vi "Emballage_BDD_CreationRapportParCarton_Modele.vi"(8 "error in (no error)":errorcluster caption="entrée d'erreur (pas d'erreur)", 11 "N° Cmd":string) -> (0 "error out":errorcluster caption="sortie d'erreur", 2 "chemin complet":path)   [LabVIEW 2020]
doc: "Envoi un mail avec la liste des valves emballées en pièce jointe si spécifié dans le fichier XML PP de la valve (FlatProp) ou correspondance produit code barre.txt (autres valves)"
uses:
  Modules/FS/60_FS_Controles/60_FS_SetGet.ctl
panel:
  out "temps Exe [s] 1":dbl
  out "temps Exe [s]":dbl
  out "Liste n° pièces de la cmde":string[](array[string])
  out "Carton":string[](array[string])
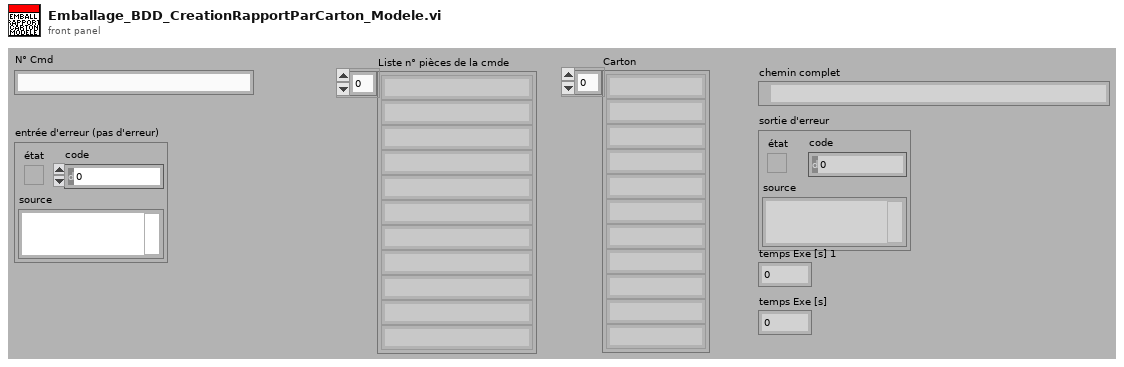
[diagram p1: front panel]
types:
  T1 = typedef "60_FS_SetGet.ctl" = enum16{"set", "get"}
  T2 = typedef "DATA commande.ctl" = cluster{"n°article FAS":string, "n° cmde FAS":string, "quantité cmde":string, "ID LIG cmde":string, "n° cmde client":string, "nom client":string, "n° article client":string, "indice revision client":string, "société de facturation":string, "langue a utiliser":string}
  T3 = cluster{"Admin-réseau":path, "XML-Réseau":path, " Résultat tests-Réseau":path, " Archive prôbleme-Réseau":path, " Archive Test  Local":path}
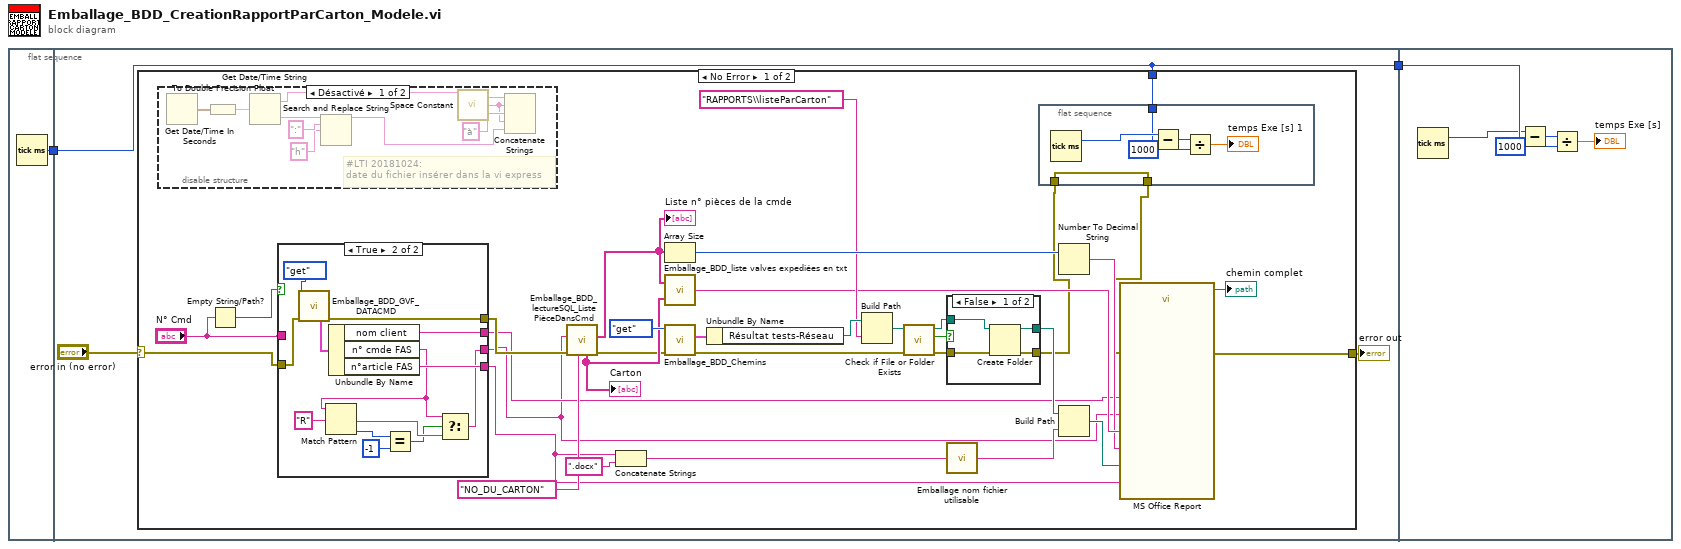
[diagram p0: block diagram]
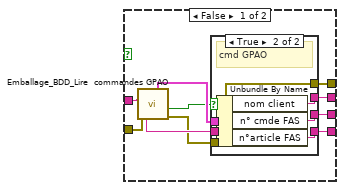
[diagram p2: hidden frame]
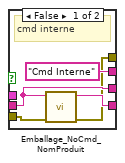
[diagram p3: hidden frame]
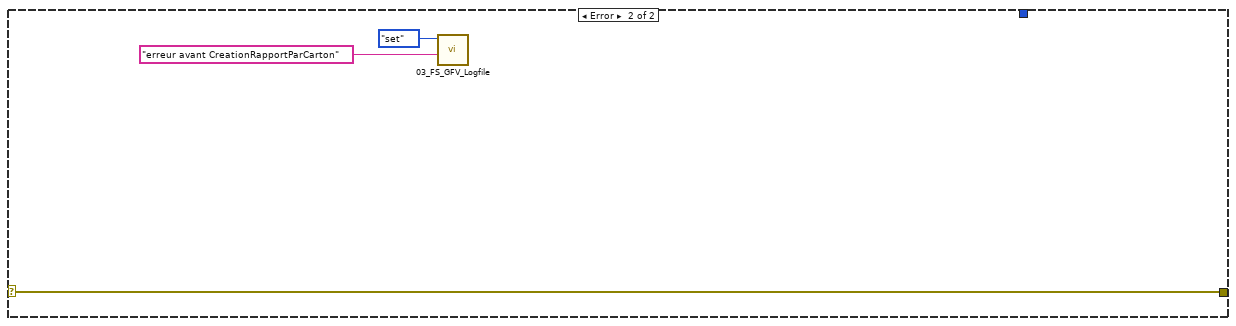
[diagram p6: hidden frame]
diagram:
  n1 = flat-sequence {
    tunnel: [w3] -> w2
    tunnel: w2 -> [w4]
    tunnel: [w4] -> w1
    tunnel: w1 -> [w100]
    frame #0 {
      n2 = Tick Count (ms)() -> (millisecond timer value=w3:u32)
    }
    frame #1 {
      n3 = case shown="No Error" "error in (no error)" {
        selector: "error in (no error)" -> [w11 w95]
        tunnel: [w19 w95] -> w5
        tunnel: w4 -> [w17 _]
        frame No Error {
          n4 = disable-structure shown="Désactivé" {
            frame Disabled {
              # "#LTI 20181024:\ndate du fichier insérer dans la vi express"
              n5 = Get Date/Time In Seconds() -> (seconds since 1Jan1904=w85:timestamp)
              n6 = To Double Precision Float(number=w85) -> (double precision float=w86:dbl)
              n7 = Get Date/Time String(seconds (now)=w86) -> (date string=w79:string, time string=w82:string)  [unwired: 2 in]
              n8 = Search and Replace String(input string=w82, search string=":" ("chaîne recherchée"), replace string="h" ("chaîne de remplacement (\"\")")) -> (result string=w80:string)  [unwired: 5 in, 3 out]
              n9 = call <vilib>:"Space Constant.vi"() -> ("String"=w78:string)
              n10 = Concatenate Strings(w79, w78, "à" ("chaîne"), w78, w80) -> ()  [unwired: 1 out]
            }
            frame Enabled {
            }
          }
          n11 = Empty String/Path?(string/path="N° Cmd") -> (empty?=w12:bool)
          n12 = case shown="True" w12 {
            tunnel: w11 -> [w48 w69]
            tunnel: [w40 w68] -> w10
            tunnel: [w45 w61] -> w7
            tunnel: [w47 w67] -> w9
            tunnel: [w46 w59] -> w8
            tunnel: "N° Cmd" -> [w42 _]
            frame False {
              n13 = call "Emballage_BDD_Lire  commandes GPAO.vi"("error in"=w48, "Numéro commande"=w42) -> ("error out"=w41:errorcluster, "existe ?"=w43:bool, "DATA cmde"=w44:T2)  [unwired: 4 in, 3 out]
              n14 = case shown="True" w43 {
                tunnel: ["Cmd Interne" ("nom client") w58] -> w47
                tunnel: [w52 w57] -> w46
                tunnel: [w51 w56] -> w45
                tunnel: w44 -> [_ w55]
                tunnel: w42 -> [w52 _]
                tunnel: w41 -> [w50 w54]
                tunnel: [w49 w54] -> w40
                frame False {
                  # "cmd interne"
                  n15 = call "Emballage_NoCmd_NomProduit.vi"("Error in"=w50, "NO_CDEVAL"=w52) -> ("Error out"=w49:errorcluster, "Produit"=w51:string)  [unwired: 8 in]
                }
                frame True {
                  # "cmd GPAO"
                  n16 = Unbundle By Name(w55) -> ("nom client"=w58:string, "n° cmde FAS"=w57:string, "n°article FAS"=w56:string)
                }
              }
            }
            frame True {
              n17 = call "Emballage_BDD_GVF_DATACMD.vi"("SetGet"=60_FS_SetGet."get", "Error in"=w69) -> ("DATA cmde OUT"=w70:T2, "Error out"=w68:errorcluster)  [unwired: 6 in, 6 out]
              n18 = Unbundle By Name(w70) -> ("nom client"=w67:string, "n° cmde FAS"=w60:string, "n°article FAS"=w61:string)
              n19 = Match Pattern(string=w60, regular expression="R" ("expression régulière")) -> (after substring=w64:string, offset past match=w63:i32)  [unwired: 1 in, 2 out]
              n20 = Equal?(x=w63, y=-1) -> (x = y?=w62:bool)
              n21 = Select(t=w60, s=w62, f=w64) -> (s? t:f=w59:string)
            }
          }
          n22 = call "Emballage_BDD_lectureSQL_Liste PièceDansCmd.vi"("order by"="NO_DU_CARTON", "Error in"=w10, "NO_CDEVAL"=w8) -> ("Error out"=w25:errorcluster, "Liste n° pièces de la cmde"=w26:string[], "Carton"=w27:string[])  [unwired: 4 in, 2 out]
          "Carton" <- w27
          "Liste n° pièces de la cmde" <- w26
          n23 = Concatenate Strings(w7, ".docx" ("chaîne")) -> (w38:string)
          n24 = Array Size(array=w26) -> (size(s)=w39:i32)
          n25 = call "Emballage_BDD_liste valves expediées en txt.vi"("Carton"=w27, "Liste n° pièces de la cmde"=w26) -> ("liste valves"=w22:string)
          n26 = call "Emballage_BDD_Chemins.vi"("error in (no error)"=w25, "SetGet"=60_FS_SetGet."get") -> ("error out"=w24:errorcluster, "CLT_Chemins_out"=w32:T3)  [unwired: 8 in]
          n27 = Unbundle By Name(w32) -> ("Résultat tests-Réseau"=w31:path)
          n28 = Build Path(base path=w31, name or relative path="RAPPORTS\\listeParCarton" ("chemin local RELEVES AUTOM\\EMBALL_...")) -> (appended path=w29:path)
          n29 = call <vilib>:"Check if File or Folder Exists.vi"("error in (no error)"=w24, "path"=w29) -> ("error out"=w35:errorcluster, "file or folder exists?"=w36:bool, "dup path"=w34:path)  [unwired: 7 in]
          n30 = case shown="False" w36 {
            tunnel: [w87 w92] -> w15
            tunnel: w35 -> [w90 w92]
            tunnel: w34 -> [w89 w91]
            tunnel: [w88 w91] -> w33
            frame False {
              n31 = Create Folder(path (use dialog)=w89, error in=w90) -> (created path=w88:path, error out=w87:errorcluster)  [unwired: 1 in, 1 out]
            }
            frame True {
            }
          }
          n32 = call "Emballage nom fichier utilisable.vi"("chaîne en entrée"=w38) -> ("chaîne résultante"=w37:string)
          n33 = flat-sequence {
            tunnel: w17 -> [w73]
            tunnel: [w72] -> w16
            tunnel: w15 -> [w72]
            frame #0 {
              n34 = Tick Count (ms)() -> (millisecond timer value=w77:u32)
              n35 = Subtract(x=w77, y=w73) -> (x-y=w74:u32)
              n36 = Divide(x=w74, y=u32 1000) -> (x/y=→"temps Exe [s] 1":dbl)
            }
          }
          n37 = Number To Decimal String(number=w39) -> (decimal integer string=w20:string)  [unwired: 1 in]
          n38 = Build Path(base path=w33, name or relative path=w37) -> (appended path=w21:path)
          n39 = call "MS Office Report"("Path to Save Report"=w21, "Client"=w9, "Commande"=w8, "Liste"=w22, "NbValvesTotal"=w20, "Produit"=w7, "error in (no error)"=w16) -> ("Saved Report Path"=→"chemin complet":path, "error out"=w19:errorcluster)  [unwired: 19 in]
        }
        frame Error {
          n40 = call "03_FS_GFV_Logfile.vi"("Chaîne"="erreur avant CreationRapportParCarton", "States"=60_FS_SetGet."set") -> ()  [unwired: 8 in, 2 out]
        }
      }
      "error out" <- w5
    }
    frame #2 {
      n41 = Tick Count (ms)() -> (millisecond timer value=w96:u32)
      n42 = Subtract(x=w96, y=w100) -> (x-y=w99:u32)
      n43 = Divide(x=w99, y=u32 1000) -> (x/y=→"temps Exe [s]":dbl)
    }
  }
